vi "_AllThingsThingWorx.vi"   [LabVIEW 2015]
uses:
  SetServiceArrayInputs.vi
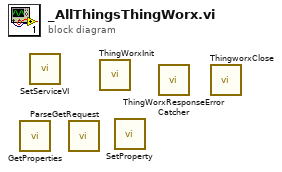
[diagram p0: block diagram]
diagram:
  n1 = call "GetProperties.vi"() -> ()  [unwired: 9 in, 3 out]
  n2 = call-poly "SetServiceVI.vi"() -> ()  [unwired: 10 in, 2 out]
  n3 = call "ParseGetRequest.vi"() -> ()  [unwired: 10 in, 2 out]
  n4 = call "ThingWorxInit.vi"() -> ()  [unwired: 10 in, 2 out]
  n5 = call "SetProperty.vi"() -> ()  [unwired: 10 in, 2 out]
  n6 = call "ThingWorxResponseErrorCatcher.vi"() -> ()  [unwired: 11 in, 1 out]
  n7 = call "ThingworxClose.vi"() -> ()  [unwired: 5 in, 1 out]
